vi "in_all i not equal to j.vi"(10 "index":i32, 11 "N":i32) -> (3 "index values":i32[](array[numeric]))   [LabVIEW 2017, in "NI_Gmath.lvlib"]
uses:
  <vilib>/gmath/NI_Gmath.lvlib
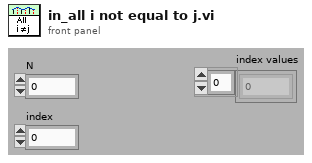
[diagram p1: front panel]
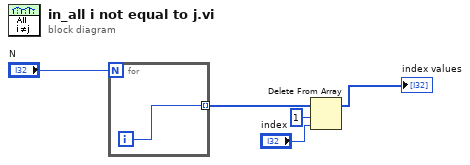
[diagram p0: block diagram]
diagram:
  n1 = for {
    N: "N" -> [_]
    tunnel: [w6] -> w4 mode=indexing
    i -> [w6]
  }
  n2 = Delete From Array(array=w4, length=1, index="index") -> (array with subset deleted=→"index values":i32[])  [unwired: 1 out]
